vi "Get Roles.vi"(8 "error in (no error)":errorcluster, 11 "TestUser in":refnum<class "TestUser.lvclass">) -> (0 "error out":errorcluster, 2 "Roles":string[](array[string]), 3 "TestUser out":refnum<class "TestUser.lvclass">)   [LabVIEW 2020, in "TestUser.lvclass"]
uses:
  TestUser.lvclass
  TestUser.lvclass/TestUser.ctl
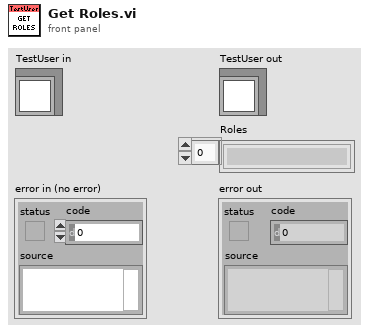
[diagram p1: front panel]
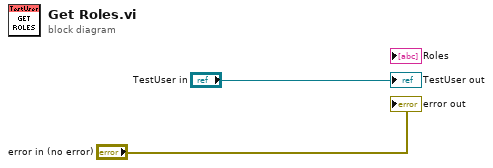
[diagram p0: block diagram]
diagram:
  "error out" <- "error in (no error)"
  "TestUser out" <- "TestUser in"
